vi "Build Log String.vi"(10 "Log Packet":T1, 11 "String Log Sink in":refnum<class "String Log Sink.lvclass">) -> (2 "Log Entry":string, 3 "String Log Sink out":refnum<class "String Log Sink.lvclass">)   [LabVIEW 2018, in "MVA Framework.lvlib" / "String Log Sink.lvclass"]
uses:
  String Log Sink.lvclass
  IStringFormat/IStringFormat.lvclass
  Composed Log/Types/Log Level.ctl
  Composed Log/Composed Log.lvlib
  Composed Log/Types/Log Packet.ctl
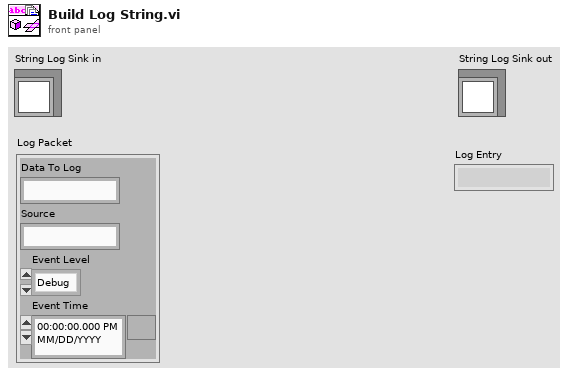
[diagram p1: front panel]
types:
  T1 = typedef "MVA Framework.lvlib/Composed Log.lvlib/Log Packet.ctl" = cluster{"Data To Log":string, "Source":string, "Event Level":T2, "Event Time":timestamp}
  T2 = typedef "MVA Framework.lvlib/Composed Log.lvlib/Log Level.ctl" = enum16{"Debug", "Info", "Warning", "Error", "Critical"}
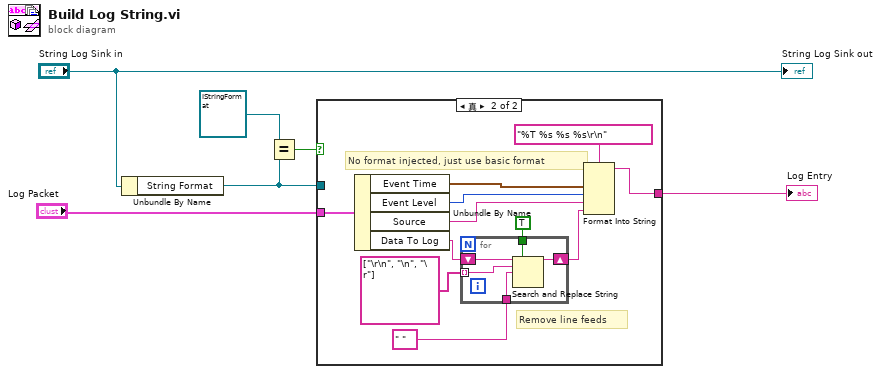
[diagram p0: block diagram]
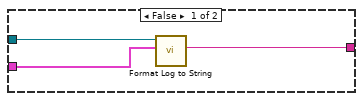
[diagram p2: hidden frame]
diagram:
  n1 = Unbundle By Name("String Log Sink in") -> ("String Format"=w4:refnum<class "IStringFormat.lvclass">)
  n2 = Equal?(x=refnum<class "IStringFormat.lvclass"> refnum ("y"), y=w4) -> (x = y?=w5:bool)
  n3 = case shown="真" w5 {
    tunnel: w4 -> [w9 _]
    tunnel: "Log Packet" -> [w8 w11]
    tunnel: [w7 w10] -> w1
    frame False {
      n4 = call-dynamic "Format Log to String.vi"("Log Packet"=w8, "IStringFormat in"=w9) -> ("Log Entry"=w7:string)  [unwired: 8 in, 1 out]
    }
    frame True {
      # "Remove line feeds"
      # "No format injected, just use basic format"
      n5 = Unbundle By Name(w11) -> ("Event Time"=w20:timestamp, "Event Level"=w18:T2, "Source"=w17:string, "Data To Log"=w16:string)
      n6 = for {
        shift-right: [w24] -> w15
        shift-left: w16 -> [w25]
        tunnel: TRUE ("replace all? (F)") -> [w23]
        tunnel: string[] ["\r\n", "\n", "\r"] ("search string") -> [w22] mode=indexing
        tunnel: " " ("replace string (\"\")") -> [w21]
        n7 = Search and Replace String(replace all?=w23, input string=w25, search string=w22, replace string=w21) -> (result string=w24:string)  [unwired: 4 in, 3 out]
      }
      n8 = Format Into String(format string="%T %s %s %s\r\n", w20, w18, w17, w15) -> (resulting string=w10:string)  [unwired: 2 in, 1 out]
    }
  }
  "Log Entry" <- w1
  "String Log Sink out" <- "String Log Sink in"
